vi "PS Serial write-read.vi"(0 "VISA Resource Name":refnum<visa-resource-name>, 5 "String To Send":string, 11 "error in (no error)":errorcluster) -> (4 "dup VISA Resource Name":refnum<visa-resource-name>, 6 "Serial Read":string, 8 "byte count":u32, 10 "Timeout":bool, 15 "error out":errorcluster)   [LabVIEW 2019]
doc: "This VI implements uses server concept for serial communication. This VI is reentrant and is an atomic read/write sequence that is guaranteed not to do another write before a read is done. This is maintained by VISA resource locking. If you want to inerleave reads and writes to the same serial port then, use the serial server VI directly which is reentrant.\nScott Hannahs <sth@magnet.fsu.edu>\nNational High Magnetic Field Lab (NHMFL)\nFlorida State University\nMay 2001"
uses:
  Serial Support VISA.llb/Serial Actions.ctl
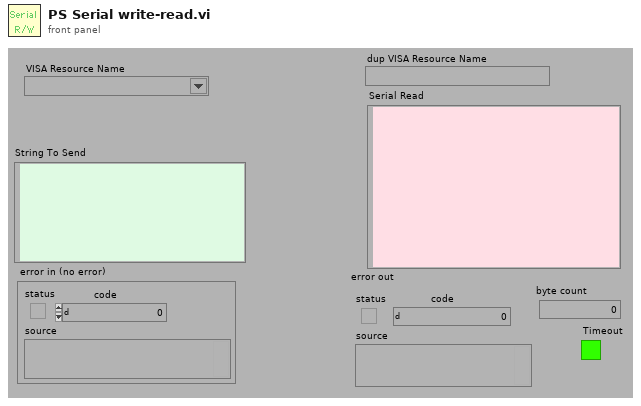
[diagram p1: front panel]
types:
  T1 = typedef "Serial Actions.ctl" = enum16{"Init", "Break", "Clear Buffer", "Write", "Read", "N Bytes", "Lock", "Unlock", "Close"}
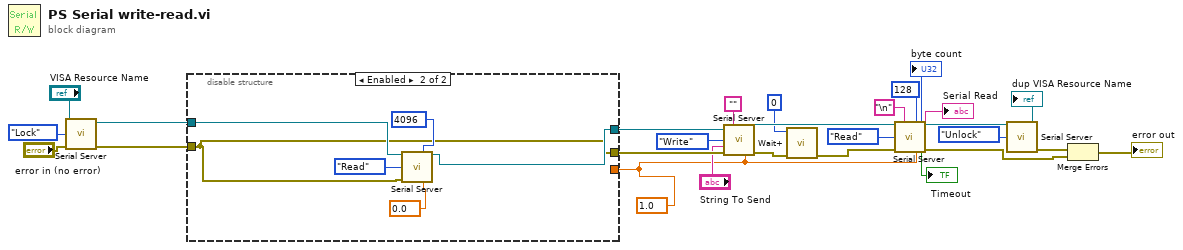
[diagram p0: block diagram]
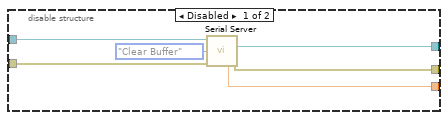
[diagram p2: hidden frame]
diagram:
  w1 = sgl 1.0 ("Timeout Limit(sec)")
  n1 = call "Serial Server.vi"("VISA Resource Name"="VISA Resource Name", "Action"=Serial_Actions."Lock", "error in (no error)"="error in (no error)") -> ("dup VISA Resource Name"=w7:refnum<visa-resource-name>, "error out"=w21:errorcluster)  [unwired: 8 in, 3 out]
  n2 = disable-structure shown="Enabled" {
    disable-tunnel: [w33 w34] -> w27
    disable-tunnel: [w32 w35] -> w26
    disable-tunnel: w21 -> [w31 w34]
    disable-tunnel: w7 -> [w29 w39]
    disable-tunnel: w1 -> [w28 _]
    frame Disabled {
      n3 = call "Serial Server.vi"("VISA Resource Name"=w29, "Action"=Serial_Actions."Clear Buffer", "error in (no error)"=w31, "Timeout Limit(sec)"=w28) -> ("dup VISA Resource Name"=w32:refnum<visa-resource-name>, "error out"=w33:errorcluster)  [unwired: 7 in, 3 out]
    }
    frame Enabled {
      n4 = call "Serial Server.vi"("VISA Resource Name"=w39, "Max Char to Read"=u32 4096, "Action"=Serial_Actions."Read", "error in (no error)"=w34, "Timeout Limit(sec)"=sgl 0.0) -> ("dup VISA Resource Name"=w35:refnum<visa-resource-name>)  [unwired: 6 in, 4 out]
    }
  }
  n5 = call "Serial Server.vi"("VISA Resource Name"=w26, "EOT Chars (cr/lf)"="", "Action"=Serial_Actions."Write", "String To Send"="String To Send", "error in (no error)"=w27, "Timeout Limit(sec)"=w1) -> ("dup VISA Resource Name"=w13:refnum<visa-resource-name>, "error out"=w12:errorcluster)  [unwired: 5 in, 3 out]
  n6 = call "Wait+.vi"("Error In"=w12, "milliseconds to wait"=u32 0) -> ("Error Out"=w6:errorcluster)  [unwired: 4 in, 1 out]
  n7 = call "Serial Server.vi"("VISA Resource Name"=w13, "EOT Chars (cr/lf)"="\n", "Max Char to Read"=u32 128, "Action"=Serial_Actions."Read", "error in (no error)"=w6, "Timeout Limit(sec)"=w1) -> ("dup VISA Resource Name"=w18:refnum<visa-resource-name>, "byte count"=→"byte count":u32, "Serial Read"=→"Serial Read":string, "Timeout"=→"Timeout":bool, "error out"=w3:errorcluster)  [unwired: 5 in]
  n8 = call "Serial Server.vi"("VISA Resource Name"=w18, "Action"=Serial_Actions."Unlock") -> ("dup VISA Resource Name"=→"dup VISA Resource Name":refnum<visa-resource-name>, "error out"=w4:errorcluster)  [unwired: 9 in, 3 out]
  n9 = Merge Errors(w4, w3) -> (→"error out":errorcluster)
